vi "configure.vi"(8 "error in (no error)":errorcluster, 9 "Value":i32, 10 "ILC":refnum<class "ILC.lvclass">, 11 "IConfigureILCStrategy in":refnum<class "ConfigureILCDAC1Strategy.lvclass">) -> (0 "error out":errorcluster, 2 "ILC 2":refnum<class "ILC.lvclass">, 3 "IConfigureILCStrategy out":refnum<class "ConfigureILCDAC1Strategy.lvclass">)   [LabVIEW 2015, in "ConfigureILCDAC1Strategy.lvclass"]
uses:
  ConfigureILCDAC1Strategy.lvclass
  <userlib>/Common/ILC/ILC/ILC.lvclass
  <userlib>/Common/ILC/ILC/ILC.lvclass/ILC.ctl
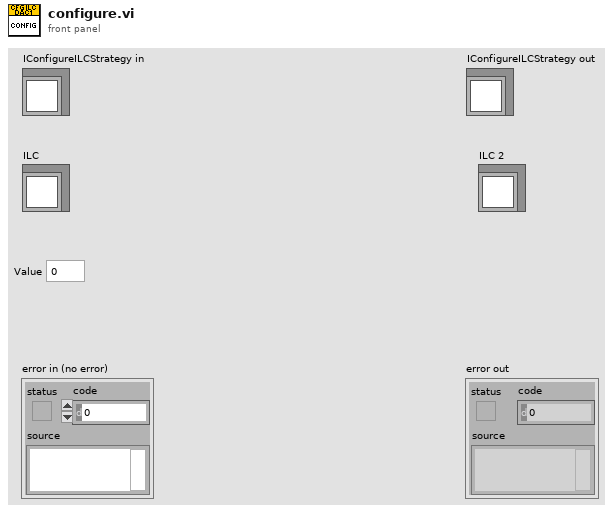
[diagram p1: front panel]
types:
  T1 = typedef "ILCCommon.lvlib/ILCTypedefs.lvlib/Outputs.ctl" = cluster{"Step & Direction":i16, "Blower RPM":u8, "PWM (SSR)":u8, "Ch1":u16, "Ch2":u16, "Ch3":u16, "Ch4":u16}
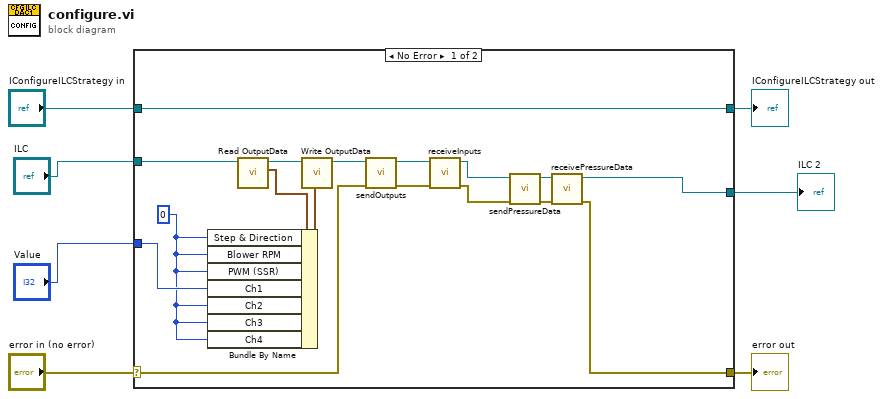
[diagram p0: block diagram]
diagram:
  n1 = case shown="No Error" "error in (no error)" {
    selector: "error in (no error)" -> [w16 w27]
    tunnel: [w8 w27] -> w6
    tunnel: [w24 w26] -> w4
    tunnel: "IConfigureILCStrategy in" -> [w24 w26]
    tunnel: "ILC" -> [w23 w25]
    tunnel: "Value" -> [w21 _]
    tunnel: [w10 w25] -> w1
    frame No Error {
      w14 = i16 0 ("Step & Direction")
      n2 = call <userlib>:"Read OutputData.vi"("ILC in"=w23) -> ("OutputData"=w22:T1, "ILC out"=w19:refnum<class "ILC.lvclass">)  [unwired: 9 in]
      n3 = Bundle By Name(cluster=w22, "Step & Direction"=w14, "Blower RPM"=w14, "PWM (SSR)"=w14, "Ch1"=w21, "Ch2"=w14, "Ch3"=w14, "Ch4"=w14) -> (w20:T1)
      n4 = call <userlib>:"Write OutputData.vi"("OutputData"=w20, "ILC in"=w19) -> ("ILC out"=w18:refnum<class "ILC.lvclass">)  [unwired: 9 in]
      n5 = call <userlib>:"sendOutputs.vi"("error in (no error)"=w16, "ILC in"=w18) -> ("error out"=w15:errorcluster, "ILC out"=w17:refnum<class "ILC.lvclass">)  [unwired: 8 in]
      n6 = call <userlib>:"receiveInputs.vi"("error in (no error)"=w15, "ILC in"=w17) -> ("error out"=w9:errorcluster, "ILC out"=w11:refnum<class "ILC.lvclass">)  [unwired: 6 in, 2 out]
      n7 = call <userlib>:"sendPressureData.vi"("error in (no error)"=w9, "ILC in"=w11) -> ("error out"=w13:errorcluster, "ILC out"=w12:refnum<class "ILC.lvclass">)  [unwired: 8 in]
      n8 = call <userlib>:"receivePressureData.vi"("error in (no error)"=w13, "ILC in"=w12) -> ("error out"=w8:errorcluster, "ILC out"=w10:refnum<class "ILC.lvclass">)  [unwired: 8 in]
    }
    frame Error {
    }
  }
  "error out" <- w6
  "IConfigureILCStrategy out" <- w4
  "ILC 2" <- w1
